vi "DHE_SetImageParams.vi"(10 "DHE_IMAGE":T1) -> ()   [LabVIEW 2016]
uses:
  private/vis/DHE_Img.ctl
  DBSHAND/private/vis/DatabaseHand_Element_Set(string).vi
  DBSHAND/private/vis/DatabaseHand_Element_Set(I32).vi
  DBSHAND/private/vis/DatabaseHand_Element_Set(bool).vi
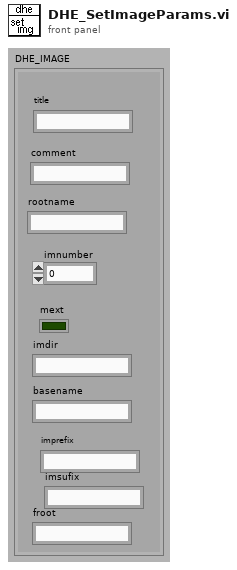
[diagram p1: front panel]
types:
  T1 = typedef "DHE_Img.ctl" = cluster{"title":string, "comment":string, "rootname":string, "imnumber":i32, "mext":bool, "imdir":string, "basename":string, "imprefix":string, "imsufix":string, "froot":string}
  T2 = typedef "DatabaseHand_RefNum.ctl" = refnum<vi>
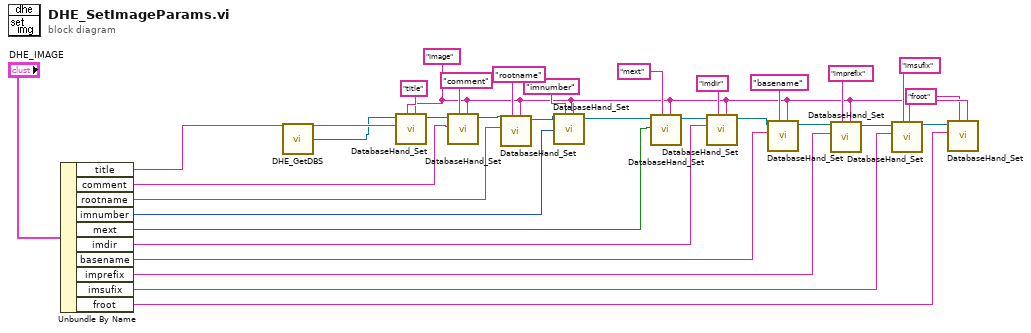
[diagram p0: block diagram]
diagram:
  w5 = "image" ("group")
  n1 = Unbundle By Name("DHE_IMAGE") -> ("title"=w31:string, "comment"=w27:string, "rootname"=w25:string, "imnumber"=w23:i32, "mext"=w19:bool, "imdir"=w9:string, "basename"=w8:string, "imprefix"=w7:string, "imsufix"=w6:string, "froot"=w2:string)
  n2 = call "DHE_GetDBS.vi"() -> ("DHE_DBSRef"=w1:T2)  [unwired: 9 out]
  n3 = call-poly "DatabaseHand_Set.vi"("group"=w5, "name"="title", "value"=w31, "Database RefNum in"=w1) -> ("Database RefNum out"=w30:T2)  [unwired: 4 in, 3 out]
  n4 = call-poly "DatabaseHand_Set.vi"("group"=w5, "name"="comment", "value"=w27, "Database RefNum in"=w30) -> ("Database RefNum out"=w29:T2)  [unwired: 4 in, 3 out]
  n5 = call-poly "DatabaseHand_Set.vi"("group"=w5, "name"="rootname", "value"=w25, "Database RefNum in"=w29) -> ("Database RefNum out"=w28:T2)  [unwired: 4 in, 3 out]
  n6 = call-poly "DatabaseHand_Set.vi"("group"=w5, "name"="imnumber", "value"=w23, "Database RefNum in"=w28) -> ("Database RefNum out"=w18:T2)  [unwired: 4 in, 3 out]
  n7 = call-poly "DatabaseHand_Set.vi"("group"=w5, "name"="mext", "value"=w19, "Database RefNum in"=w18) -> ("Database RefNum out"=w17:T2)  [unwired: 4 in, 3 out]
  n8 = call-poly "DatabaseHand_Set.vi"("group"=w5, "name"="imdir", "value"=w9, "Database RefNum in"=w17) -> ("Database RefNum out"=w16:T2)  [unwired: 4 in, 3 out]
  n9 = call-poly "DatabaseHand_Set.vi"("group"=w5, "name"="basename", "value"=w8, "Database RefNum in"=w16) -> ("Database RefNum out"=w15:T2)  [unwired: 4 in, 3 out]
  n10 = call-poly "DatabaseHand_Set.vi"("group"=w5, "name"="imprefix", "value"=w7, "Database RefNum in"=w15) -> ("Database RefNum out"=w14:T2)  [unwired: 4 in, 3 out]
  n11 = call-poly "DatabaseHand_Set.vi"("group"=w5, "name"="imsufix", "value"=w6, "Database RefNum in"=w14) -> ("Database RefNum out"=w4:T2)  [unwired: 4 in, 3 out]
  n12 = call-poly "DatabaseHand_Set.vi"("group"=w5, "name"="froot", "value"=w2, "Database RefNum in"=w4) -> ()  [unwired: 4 in, 4 out]
